vi "Toggle LED.vi"(8 "error in (no error)":errorcluster, 11 "process index":i32) -> (0 "error out":errorcluster, 3 "process index dup":i32)   [LabVIEW 2015]
doc: "Blinks the indicator."
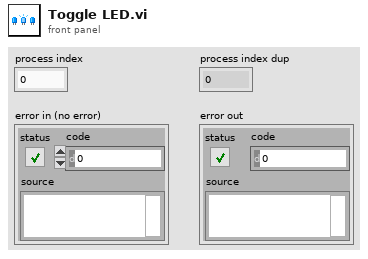
[diagram p1: front panel]
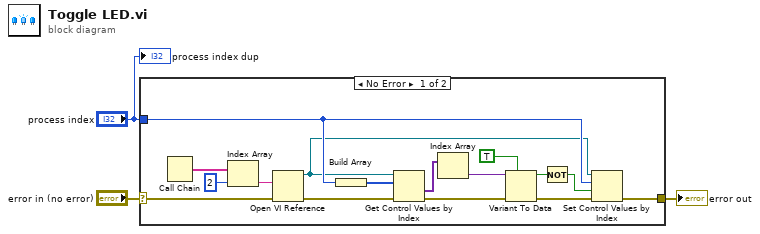
[diagram p0: block diagram]
diagram:
  n1 = case shown="No Error" "error in (no error)" {
    selector: "error in (no error)" -> [w6 w20]
    tunnel: [w19 w20] -> w3
    tunnel: "process index" -> [w15 _]
    frame No Error {
      n2 = Call Chain() -> (call chain=w7:string[])
      n3 = Index Array(array=w7, index=2) -> (element=w9:string)
      n4 = Open VI Reference(vi path=w9, error in (no error)=w6) -> (vi reference=w4:refnum<vi>, error out=w5:errorcluster)  [unwired: 4 in]
      n5 = Build Array(w15) -> (w10:i32[])
      n6 = Get Control Values by Index(0:w4, 1:w10, 3:w5) -> (10:w11:variant[], 11:w18:errorcluster)
      n7 = Index Array(array=w11) -> (element=w12:variant)  [unwired: 1 in]
      n8 = Variant To Data(error in=w18, type=TRUE, Variant=w12) -> (data=w14:bool, error out=w17:errorcluster)
      n9 = Not(x=w14) -> (.not. x?=w16:bool)
      n10 = Set Control Values by Index(0:w4, 1:w15, 2:w16, 3:w17) -> (11:w19:errorcluster)
    }
    frame Error {
    }
  }
  "error out" <- w3
  "process index dup" <- "process index"
